vi "MovieTemplate.vi"() -> ()   [LabVIEW 2010]
uses:
  SubVIs/LVPresent_Globals.vi
panel:
  in  "Movie Path":path=path "/Kimberly/Users/crogers/Documents/ROBOLAB Data/RoboSlides/Movies/SwissBurger.mov"
  out "Movie":picture
  # "LEGO Engineering:\nSwiss Burgers"
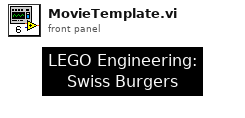
[diagram p1: front panel]
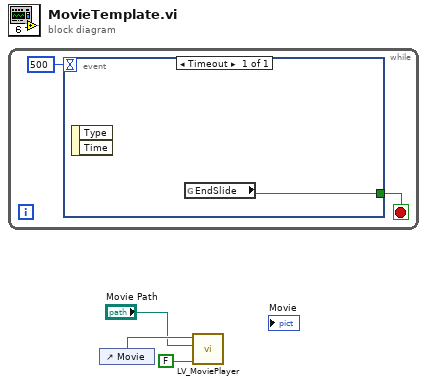
[diagram p0: block diagram]
diagram:
  n1 = while {
    stop <- w5 stop-if-true
    n2 = event shown="[0] Timeout" {
      selector: _ -> [_]
      dyn-events: _ -> [_]
      timeout: 500 -> [_]
      tunnel: [w6] -> w5
      event Timeout {
        n3 = event-data() -> ()  [unwired: 1 in, 2 out]
        n4 = global read "LVPresent_Globals.vi" "EndSlide"() -> (w6:bool)
      }
    }
  }
  n5 = control-ref of="Movie"() -> (w3:refnum<vi>)
  n6 = call "LV_MoviePlayer.vi"("Play at maximum speed"=FALSE, "Movie Path"="Movie Path", "reference"=w3) -> ()  [unwired: 2 in, 1 out]
